vi "Build Status Tree.vi"(7 "Tree":refnum<vi>, 8 "error in (no error)":errorcluster, 11 "Volatus Core in":refnum<class "Volatus Core.lvclass">) -> (0 "error out":errorcluster, 3 "Volatus Core out":refnum<class "Volatus Core.lvclass">)   [LabVIEW 2020, in "Volatus.lvlib" / "Volatus Core.lvclass"]
uses:
  Volatus Core.lvclass
  Volatus Core.lvclass/Volatus Core.ctl
  lv-tree-tools/Tree Map/Tree Map/Tree Map.lvclass
  lv-tree-tools/Tree Map/Tree Map/Extra Entry Info.ctl
panel:
  out "error out 2":errorcluster
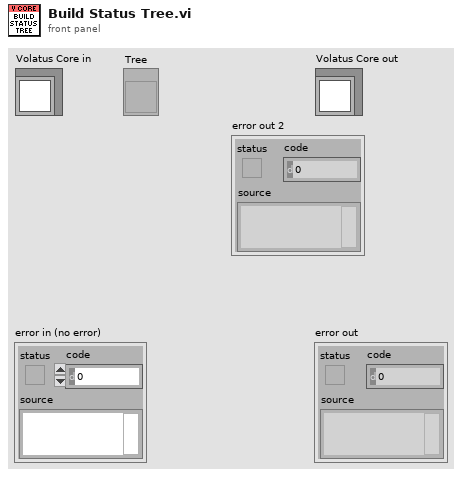
[diagram p1: front panel]
types:
  T1 = typedef "Volatus.lvlib/Module Status.ctl" = cluster{"Hierarchy":string[], "State":T2, "Substatus":map{string, string}, "Metrics":map{string, dbl}}
  T2 = typedef "Volatus.lvlib/Module.lvclass/State.ctl" = enum16{"Unknown", "Launched", "Starting", "Running", "Stopping", "Stopped", "Error - Starting", "Error - Run", "Error - Stopping"}
  T3 = typedef "Tree Map.lvlib/Tree Map.lvclass/Extra Entry Info.ctl" = cluster{"BG Color":u32, "Symbol":i32}
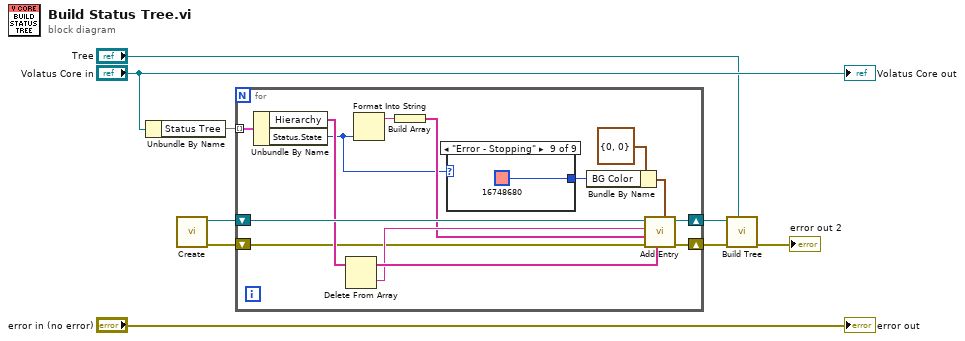
[diagram p0: block diagram]
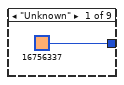
[diagram p2: hidden frame]
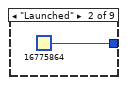
[diagram p3: hidden frame]
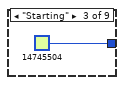
[diagram p4: hidden frame]
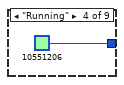
[diagram p5: hidden frame]
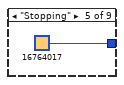
[diagram p6: hidden frame]
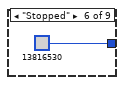
[diagram p7: hidden frame]
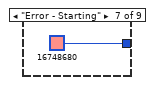
[diagram p8: hidden frame]
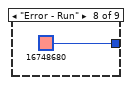
[diagram p9: hidden frame]
diagram:
  n1 = Unbundle By Name("Volatus Core in") -> ("Status Tree"=w7:map{string[], T1})
  n2 = call "Create.vi"() -> ("error out"=w3:errorcluster, "Tree Map out"=w6:refnum<class "Tree Map.lvclass">)  [unwired: 10 in]
  n3 = for {
    tunnel: w7 -> [w23] mode=indexing
    shift-right: [w18] -> w5
    shift-left: w6 -> [w22]
    shift-right: [w14] -> w2
    shift-left: w3 -> [w15]
    n4 = Unbundle By Name(w23) -> ("Hierarchy"=w21:string[], "Status.State"=w13:T2)
    n5 = Delete From Array(array=w21) -> (deleted portion=w19:string, array with subset deleted=w20:string[])  [unwired: 2 in]
    n6 = Format Into String(w13) -> (resulting string=w17:string)  [unwired: 3 in, 1 out]
    n7 = Build Array(w17) -> (w16:string[])
    n8 = case shown="\"Error - Stopping\"" w13 {
      tunnel: [u32 16756337 u32 16775864 u32 14745504 u32 10551206 u32 16764017 u32 13816530 u32 16748680 u32 16748680 u32 16748680] -> w11
      frame "Unknown" {
      }
      frame "Launched" {
      }
      frame "Starting" {
      }
      frame "Running" {
      }
      frame "Stopping" {
      }
      frame "Stopped" {
      }
      frame "Error - Starting" {
      }
      frame "Error - Run" {
      }
      frame "Error - Stopping" {
      }
    }
    n9 = Bundle By Name(cluster=T3 {"BG Color"=0, "Symbol"=0} ("Extra Info"), "BG Color"=w11) -> (w10:T3)
    n10 = call "Add Entry.vi"("Extra Info"=w10, "Parent (None)"=w20, "error in (no error)"=w15, "Columns"=w16, "Name"=w19, "Tree Map in"=w22) -> ("error out"=w14:errorcluster, "Tree Map out"=w18:refnum<class "Tree Map.lvclass">)  [unwired: 3 in, 1 out]
  }
  n11 = call "Build Tree.vi"("Tree"="Tree", "error in (no error)"=w2, "Tree Map in"=w5) -> ("error out"=→"error out 2":errorcluster)  [unwired: 7 in, 1 out]
  "error out" <- "error in (no error)"
  "Volatus Core out" <- "Volatus Core in"
